vi "file viewer_ calibration attempt.vi"() -> ()   [LabVIEW 2017]
uses:
  <vilib>/Utility/file.llb/Read Delimited Spreadsheet (I64).vi
  <vilib>/Analysis/NI_AALPro.lvlib
panel:
  out "HHG order":dbl
  in  "X":dbl
  out "XY Graph":T1(graph)
  in  "Array":dbl[][](array[numeric])
  out "Pixel Row":i64[](graph)
  in  "Y pixel position":dbl
  in  "file path for picture":path
  in  "?":bool
  out "Intensity Graph":i32[][](graph)
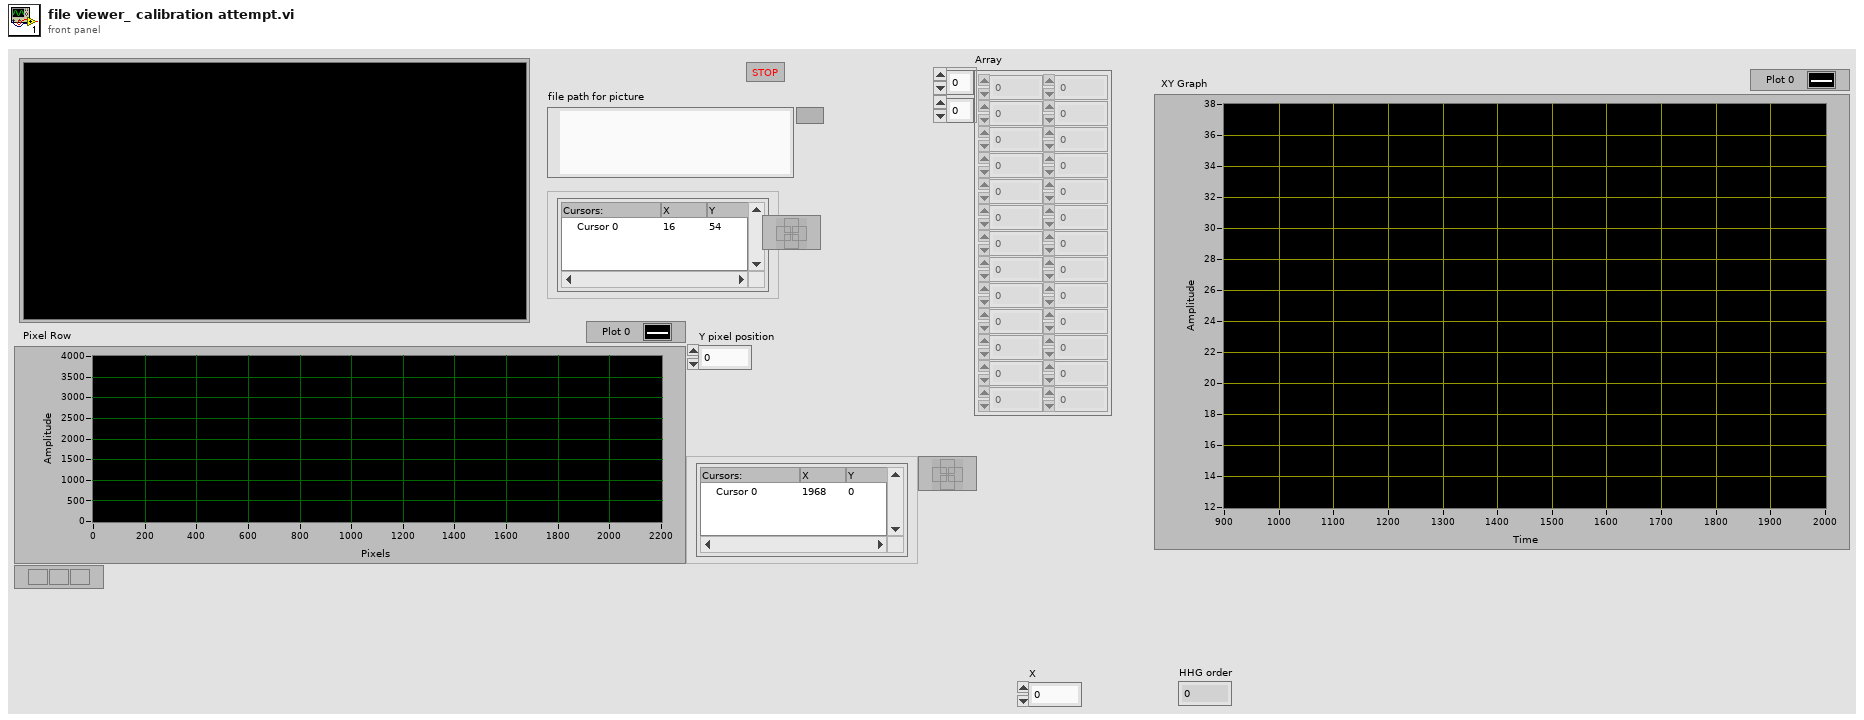
[diagram p1: front panel]
types:
  T1 = cluster{"Array":dbl[], "Best Polynomial Fit":dbl[]}[]
  T2 = cluster{"Array":dbl[], "Best Polynomial Fit":dbl[]}
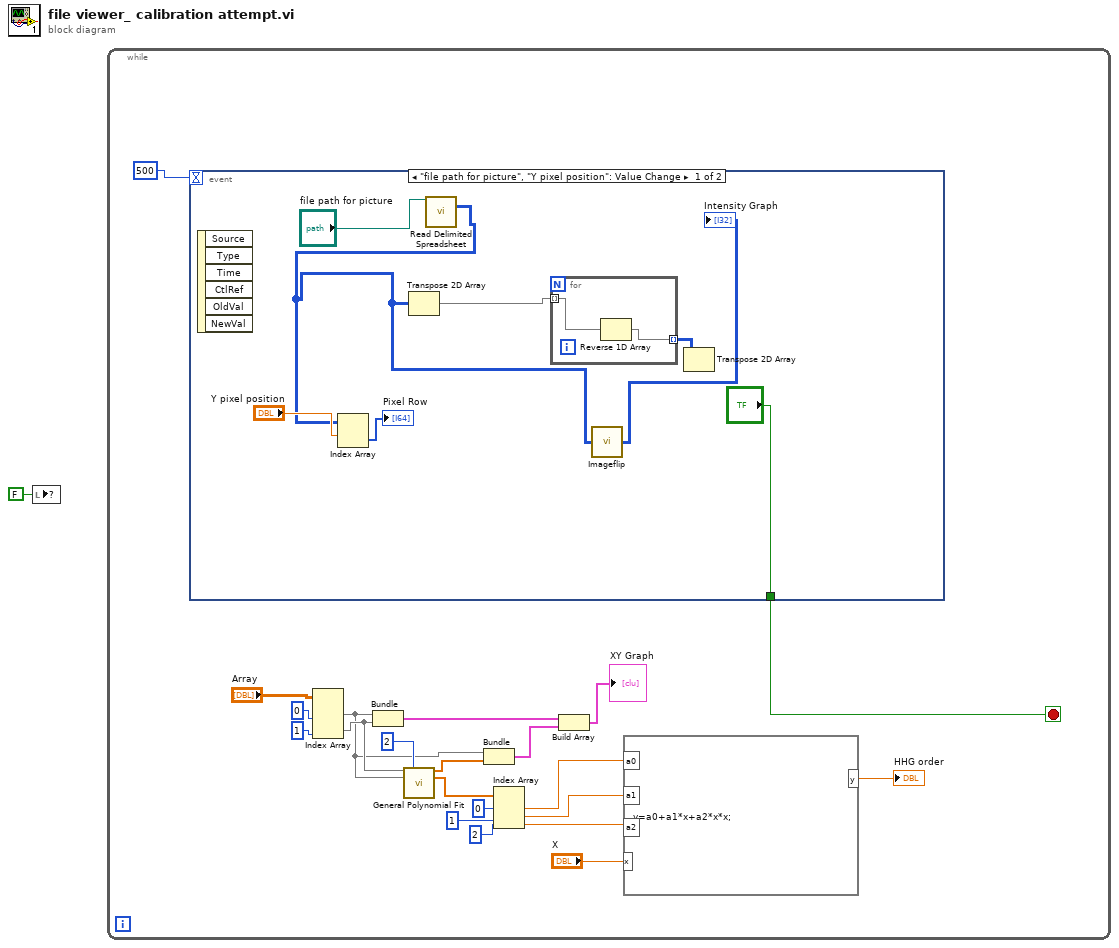
[diagram p0: block diagram]
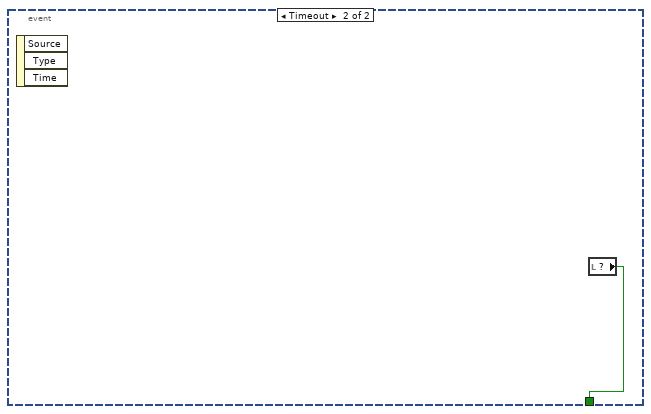
[diagram p2: hidden frame]
diagram:
  n1 = local write item#1(FALSE) -> ()
  n2 = while {
    stop <- w22 stop-if-true
    n3 = event shown="[0] \"file path for picture\", \"Y pixel position\": Value Change" {
      selector: _ -> [_ _]
      dyn-events: _ -> [_ _]
      timeout: 500 -> [_ _]
      tunnel: ["?" w33] -> w22
      event "file path for picture", "Y pixel position": Value Change {
        n4 = event-data() -> ()  [unwired: 1 in, 6 out]
        n5 = call-poly <vilib>:"Read Delimited Spreadsheet.vi"("file path (dialog if empty)"="file path for picture") -> ("all rows"=w24:i64[][])  [unwired: 9 in, 5 out]
        n6 = Index Array(array=w24, index (row)="Y pixel position") -> (element=→"Pixel Row":i64[])  [unwired: 1 in]
        n7 = Transpose 2D Array(2D array=w24) -> (transposed array=w26:i64[][])
        n8 = for {
          tunnel: w26 -> [w32] mode=indexing
          tunnel: [w31] -> w25 mode=indexing
          n9 = Reverse 1D Array(array=w32) -> (reversed array=w31:i64[])
        }
        n10 = call "Imageflip.vi"("2D array"=w24) -> ("transposed array"=→"Intensity Graph":i32[][])
        n11 = Transpose 2D Array(2D array=w25) -> ()  [unwired: 1 out]
      }
      event Timeout {
        n12 = event-data() -> ()  [unwired: 1 in, 3 out]
        n13 = local read item#1() -> (w33:bool)
      }
    }
    n14 = Index Array(array="Array", index (col) #1=0 ("index"), index (col) #2=1 ("index")) -> (element #1=w11:dbl[], element #2=w15:dbl[])  [unwired: 2 in]
    n15 = Bundle("Array"=w11, "Array"=w15) -> (w13:cluster{"Array":dbl[], "Array":dbl[]})  [unwired: 1 in]
    n16 = call <vilib>:"General Polynomial Fit.vi"("Y"=w15, "polynomial order"=2, "X"=w11) -> ("Best Polynomial Fit"=w16:dbl[], "Polynomial Coefficients"=w10:dbl[])  [unwired: 9 in, 2 out]
    n17 = Bundle("Array"=w11, "Best Polynomial Fit"=w16) -> (w14:T2)  [unwired: 1 in]
    n18 = Index Array(array=w10, index #1=0 ("index"), index #2=1 ("index"), index #3=2 ("index")) -> (element #1=w6:dbl, element #2=w5:dbl, element #3=w4:dbl)
    n19 = Build Array(w13, w14) -> (→"XY Graph":T1)
    n20 = formula code="y=a0+a1*x+a2*x*x;"("a0"=w6, "a1"=w5, "a2"=w4, "x"="X") -> ("y"=→"HHG order":dbl)
  }
